vi "palindrome using strings.vi"() -> ()   [LabVIEW 2018]
panel:
  out "String":string
  in  "string":string
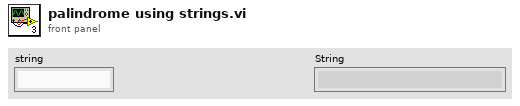
[diagram p1: front panel]
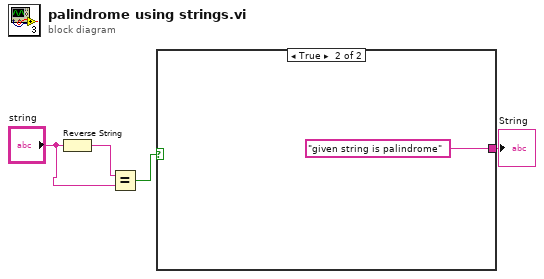
[diagram p0: block diagram]
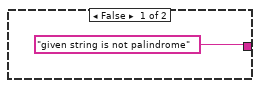
[diagram p2: hidden frame]
diagram:
  n1 = Reverse String(1:"string") -> (0:w4:string)
  n2 = Equal?(x=w4, y="string") -> (x = y?=w3:bool)
  n3 = case shown="True" w3 {
    tunnel: ["given string is not palindrome" "given string is palindrome"] -> w2
    frame False {
    }
    frame True {
    }
  }
  "String" <- w2
